vi "turnEncoder.vi"(8 "speed (%)":dbl, 9 "angle (right)":dbl, 10 "rightMotor":T1={"DeviceStatus"={"status"=FALSE, "code"=0, "source"=""}, "Type"=enum."PWM", "PWM"={"PWM Channel"=enum."Invalid", "DeadBand"={"Name"="", "maxPositivePwm"=0, "minPositivePwm"=0, "centerPwm"=0, "maxNegativePwm"=0, "minNegativePwm"=0, "angularRange"=0}}, "CAN"={"Device Number"=0, "SetOutput VI Ref"=variant(refnum<vi> refnum), "GetOutput VI Ref"=variant(refnum<vi> refnum), "Enable VI Ref"=variant(refnum<vi> refnum), "Disable VI Ref"=variant(refnum<vi> refnum), "Data"=variant}, "Invert"=FALSE}, 11 "leftMotor":T1={"DeviceStatus"={"status"=FALSE, "code"=0, "source"=""}, "Type"=enum."PWM", "PWM"={"PWM Channel"=enum."Invalid", "DeadBand"={"Name"="", "maxPositivePwm"=0, "minPositivePwm"=0, "centerPwm"=0, "maxNegativePwm"=0, "minNegativePwm"=0, "angularRange"=0}}, "CAN"={"Device Number"=0, "SetOutput VI Ref"=variant(refnum<vi> refnum), "GetOutput VI Ref"=variant(refnum<vi> refnum), "Enable VI Ref"=variant(refnum<vi> refnum), "Disable VI Ref"=variant(refnum<vi> refnum), "Data"=variant}, "Invert"=FALSE}) -> (2 "rightMotor":T1={"DeviceStatus"={"status"=FALSE, "code"=0, "source"=""}, "Type"=enum."PWM", "PWM"={"PWM Channel"=enum."Invalid", "DeadBand"={"Name"="", "maxPositivePwm"=0, "minPositivePwm"=0, "centerPwm"=0, "maxNegativePwm"=0, "minNegativePwm"=0, "angularRange"=0}}, "CAN"={"Device Number"=0, "SetOutput VI Ref"=variant(enum8{"Percent VBus", "Current", "Speed", "Position", "Voltage"} enum."Percent VBus"), "GetOutput VI Ref"=variant(refnum<k1> refnum), "Enable VI Ref"=variant(dbl 12.0), "Disable VI Ref"=variant(enum8{"Percent VBus", "Speed", "Position", "Slave", "Unchanged / Invalid"} enum."Percent VBus"), "Data"=variant}, "Invert"=FALSE}, 3 "leftMotor":T1={"DeviceStatus"={"status"=FALSE, "code"=0, "source"=""}, "Type"=enum."PWM", "PWM"={"PWM Channel"=enum."Invalid", "DeadBand"={"Name"="", "maxPositivePwm"=0, "minPositivePwm"=0, "centerPwm"=0, "maxNegativePwm"=0, "minNegativePwm"=0, "angularRange"=0}}, "CAN"={"Device Number"=0, "SetOutput VI Ref"=variant(enum8{"Percent VBus", "Current", "Speed", "Position", "Voltage"} enum."Percent VBus"), "GetOutput VI Ref"=variant(refnum<k1> refnum), "Enable VI Ref"=variant(dbl 12.0), "Disable VI Ref"=variant(enum8{"Percent VBus", "Speed", "Position", "Slave", "Unchanged / Invalid"} enum."Percent VBus"), "Data"=variant}, "Invert"=FALSE})   [LabVIEW 2016]
uses:
  <vilib>/Rock Robotics/WPI/MotorControl/WPI_MotorControlDeviceRef.ctl
  <vilib>/Rock Robotics/WPI/MotorControl/WPI_MotorControlType.ctl
  <vilib>/Rock Robotics/SystemInterfaces/DIO/FPGA_DIOPWMChannel.ctl
  <vilib>/Rock Robotics/WPI/PWM/WPI_PWMDeadband.ctl
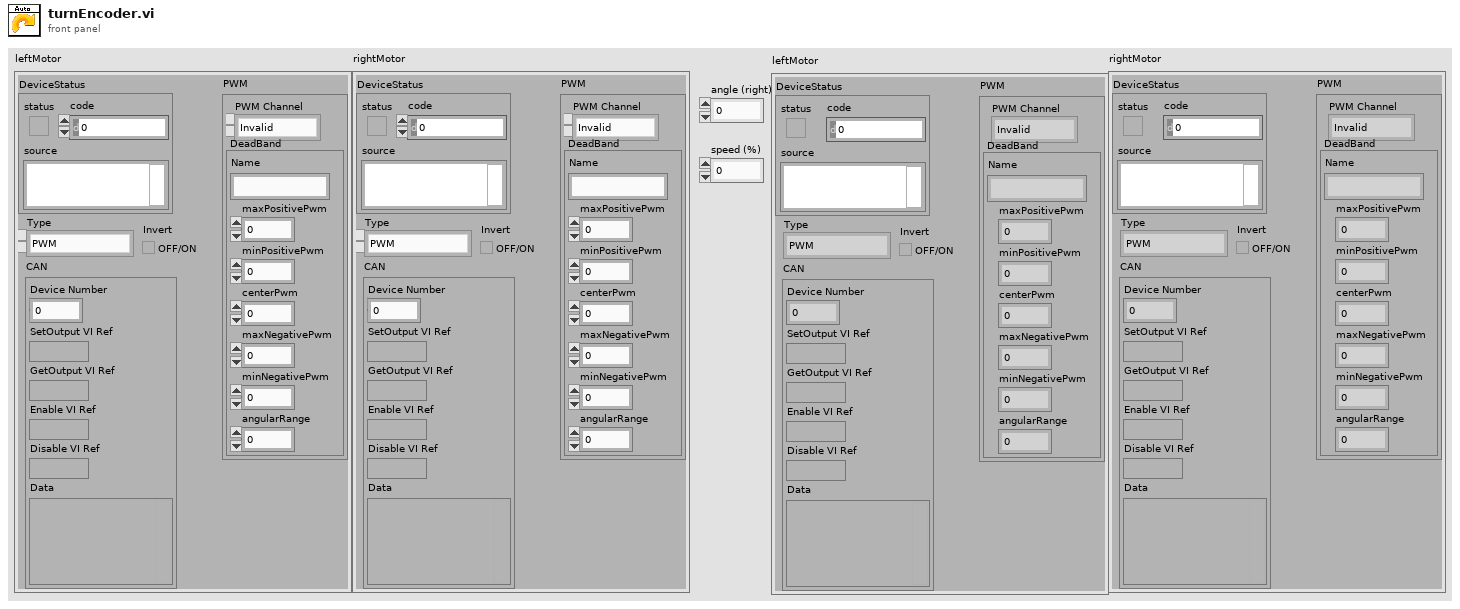
[diagram p1: front panel]
types:
  T1 = typedef "WPI_MotorControlDeviceRef.ctl" = cluster{"DeviceStatus":errorcluster, "Type":T2, "PWM":cluster{"PWM Channel":T3, "DeadBand":T4}, "CAN":cluster{"Device Number":u8, "SetOutput VI Ref":variant, "GetOutput VI Ref":variant, "Enable VI Ref":variant, "Disable VI Ref":variant, "Data":variant}, "Invert":bool}
  T2 = typedef "WPI_MotorControlType.ctl" = enum16{"PWM", "CAN"}
  T3 = typedef "FPGA_DIOPWMChannel.ctl" = enum8{"PWM 0", "PWM 1", "PWM 2", "PWM 3", "PWM 4", "PWM 5", "PWM 6", "PWM 7", "PWM 8", "PWM 9", "PWM MXP 0", "PWM MXP 1", "PWM MXP 2", "PWM MXP 3", "PWM MXP 4", "PWM MXP 5", "PWM MXP 6", "PWM MXP 7", "PWM MXP 8", "PWM MXP 9", "Invalid"}
  T4 = typedef "WPI_PWMDeadband.ctl" = cluster{"Name":string, "maxPositivePwm":i32, "minPositivePwm":i32, "centerPwm":i32, "maxNegativePwm":i32, "minNegativePwm":i32, "angularRange":u16}
  T5 = typedef "WPI_CANTalonSRX_GlobalStatus.ctl" = cluster{"Applied Throttle":dbl, "Module Enabled":bool, "CAN Error":errorcluster, "Closed Loop Error":dbl, "Forward Limit Switch Closed":bool, "Reverse Limit Switch Closed":bool, "Sensor Position":dbl, "Sensor Velocity":dbl, "Current":dbl, "Sticky Fault - Over Temp":bool, "Sticky Fault - Under Voltage":bool, "Sticky Fault - Forward Limit":bool, "Sticky Fault - Reverse Limit":bool, "Sticky Fault - Forward Soft Limit":bool, "Sticky Fault - Reverse Soft Limit":bool, "Brake is Enabled":bool, "Encoder Position":dbl, "Encoder Velocity":dbl, "Encoder Index Count":dbl, "Encoder A Pin State":bool, "Encoder B Pin State":bool, "Encoder Index Pin State":bool, "Analog In":dbl, "Analog In Velocity":dbl, "Temperature (C)":dbl, "Battery Voltage":dbl, "Control 5 Is Supported":bool, "Current Profile Slot Select":dbl, "Pos Div 8":bool, "Vel Div 4":bool, "Pulse Width Position":i32, "Pulse Width Velocity":i32, "Pulse Width Rise To Rise (us)":i32, "Pulse Width Rise To Fall (us)":i32, "Mot Prof Active Is Under Run":bool, "Mot Prof Active Has Under Run":bool, "Mot Prof Active Is Last":bool, "Mot Prof Active Velocity Only":bool, "Mot Prof Active Is Valid":bool, "Mot Prof Buffer Is Full":bool, "Mot Prof Active Profile Slot Select":i32, "Mot Prof NextID":i32, "Mot Prof Count":i32, "Mot Prof Active Velocity":dbl, "Mot Prof Active Position":dbl, "Mot Prof Output Enable":i32}
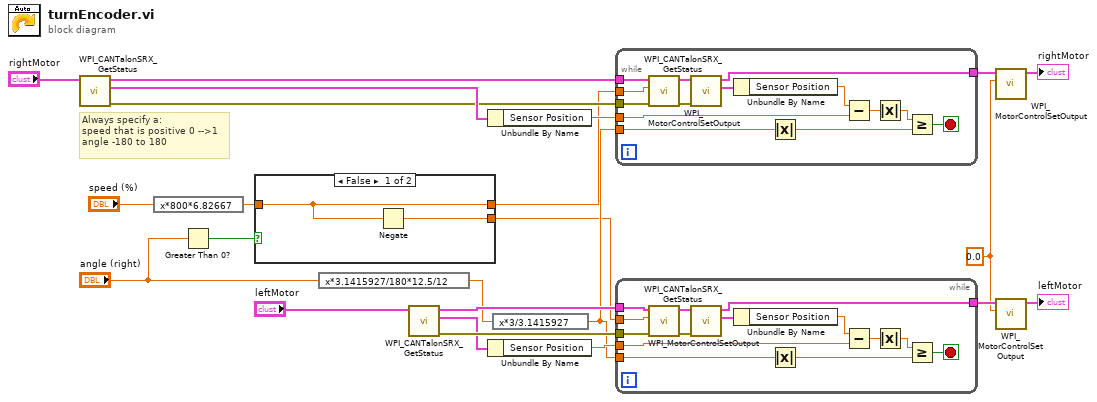
[diagram p0: block diagram]
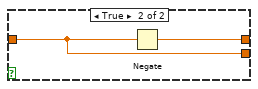
[diagram p2: hidden frame]
diagram:
  w10 = 0.0
  # "Always specify a:\nspeed that is positive 0 -->1\nangle -180 to 180"
  n1 = call <vilib>:"WPI_CANTalonSRX_GetStatus.vi"("CAN Talon SRX Ref"="rightMotor") -> ("error out"=w16:errorcluster, "Talon SRX Status"=w18:T5, "CAN Talon SRX Ref"=w17:T1)  [unwired: 8 in]
  n2 = expression code="x*800*6.82667"("speed (%)") -> (w3:dbl)
  n3 = Greater Than 0?(x="angle (right)") -> (x > 0?=w4:bool)
  n4 = case shown="False" w4 {
    tunnel: w3 -> [w24 w27]
    tunnel: [w25 w27] -> w2
    tunnel: [w24 w26] -> w1
    frame False {
      n5 = Negate(x=w24) -> (-x=w25:dbl)
    }
    frame True {
      n6 = Negate(x=w27) -> (-x=w26:dbl)
    }
  }
  n7 = expression code="x*3.1415927/180*12.5/12"("angle (right)") -> (w7:dbl)
  n8 = call <vilib>:"WPI_CANTalonSRX_GetStatus.vi"("CAN Talon SRX Ref"="leftMotor") -> ("error out"=w22:errorcluster, "Talon SRX Status"=w21:T5, "CAN Talon SRX Ref"=w23:T1)  [unwired: 8 in]
  n9 = Unbundle By Name(w18) -> ("Sensor Position"=w14:dbl)
  n10 = Unbundle By Name(w21) -> ("Sensor Position"=w19:dbl)
  n11 = expression code="x*3/3.1415927"(w7) -> (w6:dbl)
  n12 = while {
    tunnel: w17 -> [w39]
    tunnel: w16 -> [w38]
    tunnel: [w36] -> w11
    tunnel: w6 -> [w31]
    tunnel: w14 -> [w33]
    tunnel: w1 -> [w32]
    stop <- w28 stop-if-true
    n13 = call <vilib>:"WPI_MotorControlSetOutput.vi"("error in (no error)"=w38, "Output"=w32, "MotorControlDevRef"=w39) -> ("error out"=w40:errorcluster, "MotorControlDevRef"=w41:T1)  [unwired: 6 in, 1 out]
    n14 = call <vilib>:"WPI_CANTalonSRX_GetStatus.vi"("error in (no error)"=w40, "CAN Talon SRX Ref"=w41) -> ("Talon SRX Status"=w37:T5, "CAN Talon SRX Ref"=w36:T1)  [unwired: 7 in, 1 out]
    n15 = Unbundle By Name(w37) -> ("Sensor Position"=w35:dbl)
    n16 = Absolute Value(x=w31) -> (abs(x)=w29:dbl)
    n17 = Subtract(x=w35, y=w33) -> (x-y=w34:dbl)
    n18 = Absolute Value(x=w34) -> (abs(x)=w30:dbl)
    n19 = Greater Or Equal?(x=w30, y=w29) -> (x >= y?=w28:bool)
  }
  n20 = while {
    tunnel: w23 -> [w53]
    tunnel: w22 -> [w52]
    tunnel: [w50] -> w12
    tunnel: w19 -> [w48]
    tunnel: w6 -> [w45]
    tunnel: w2 -> [w46]
    stop <- w42 stop-if-true
    n21 = call <vilib>:"WPI_MotorControlSetOutput.vi"("error in (no error)"=w52, "Output"=w46, "MotorControlDevRef"=w53) -> ("error out"=w54:errorcluster, "MotorControlDevRef"=w55:T1)  [unwired: 6 in, 1 out]
    n22 = call <vilib>:"WPI_CANTalonSRX_GetStatus.vi"("error in (no error)"=w54, "CAN Talon SRX Ref"=w55) -> ("Talon SRX Status"=w51:T5, "CAN Talon SRX Ref"=w50:T1)  [unwired: 7 in, 1 out]
    n23 = Unbundle By Name(w51) -> ("Sensor Position"=w49:dbl)
    n24 = Absolute Value(x=w45) -> (abs(x)=w43:dbl)
    n25 = Subtract(x=w49, y=w48) -> (x-y=w47:dbl)
    n26 = Absolute Value(x=w47) -> (abs(x)=w44:dbl)
    n27 = Greater Or Equal?(x=w44, y=w43) -> (x >= y?=w42:bool)
  }
  n28 = call <vilib>:"WPI_MotorControlSetOutput.vi"("Output"=w10, "MotorControlDevRef"=w11) -> ("MotorControlDevRef"=→"rightMotor":T1)  [unwired: 7 in, 2 out]
  n29 = call <vilib>:"WPI_MotorControlSetOutput.vi"("Output"=w10, "MotorControlDevRef"=w12) -> ("MotorControlDevRef"=→"leftMotor":T1)  [unwired: 7 in, 2 out]
